vi "Write Tokenizer.vi"(8 "error in (no error)":errorcluster, 10 "Tokenizer":refnum<class "Lexer.lvclass">, 11 "Alpaca Parser in":refnum<class "Parser.lvclass">) -> (0 "error out":errorcluster, 3 "Alpaca Parser out":refnum<class "Parser.lvclass">)   [LabVIEW 2019, in "JKI JSON Serialization.lvlib" / "Parser.lvclass"]
doc: "JKI JSON 1.1.10.37\nTomi Maila - JKI\nCopyright (c) 2017, JKI"
uses:
  Parser.lvclass
  Lexer/Lexer.lvclass
  Parser.lvclass/Parser.ctl
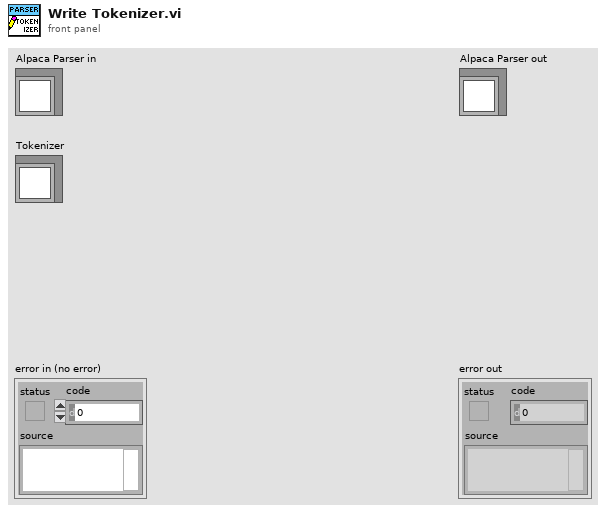
[diagram p1: front panel]
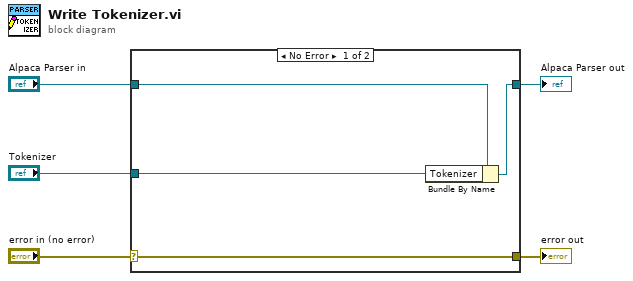
[diagram p0: block diagram]
diagram:
  n1 = case shown="No Error" "error in (no error)" {
    selector: "error in (no error)" -> [w9 w10]
    tunnel: [w9 w10] -> w4
    tunnel: [w7 w11] -> w2
    tunnel: "Alpaca Parser in" -> [w8 w11]
    tunnel: "Tokenizer" -> [w6 _]
    frame No Error {
      n2 = Bundle By Name(cluster=w8, "Tokenizer"=w6) -> (w7:refnum<class "Parser.lvclass">)
    }
    frame Error {
    }
  }
  "error out" <- w4
  "Alpaca Parser out" <- w2
